vi "enable_by_name.vi"(8 "error in (no error)":errorcluster caption="错误输入（无错误）", 10 "name":string, 11 "MotorSystem 输入":refnum<class "MotorSystem.lvclass">) -> (0 "error out":errorcluster caption="错误输出", 3 "MotorSystem 输出":refnum<class "MotorSystem.lvclass">)   [LabVIEW 2016, in "MotionControl_UFO_3DOF.lvlib" / "MotorSystem.lvclass"]
uses:
  <userlib>/MotionControl_UFO_3DOF/MotorSystem/MotorSystem.lvclass
  <userlib>/MotionControl_UFO_3DOF/MotorSystem/MotorSystem.lvclass/MotorSystem.ctl
  <userlib>/MotionControl_UFO_3DOF/OneMotion/OneMotion.lvclass
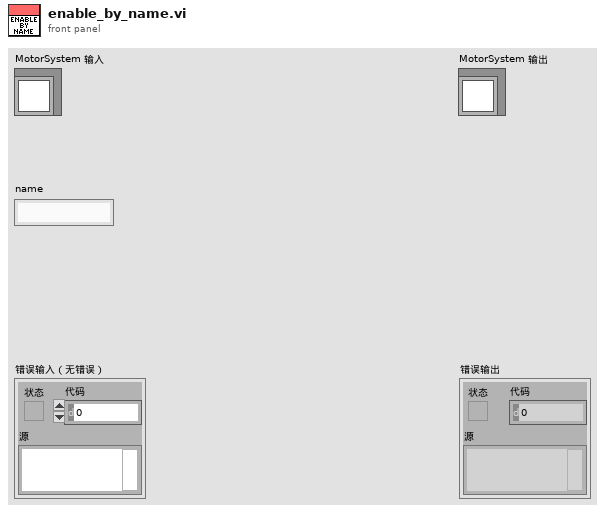
[diagram p1: front panel]
types:
  T1 = typedef "MotionControl_UFO_3DOF.lvlib/MotorSystem.lvclass/MotionCluster.ctl" = cluster{"OneMotion.lvclass":refnum<class "OneMotion.lvclass">, "connected?":bool, "default enabled?":bool, "enabled?":bool}
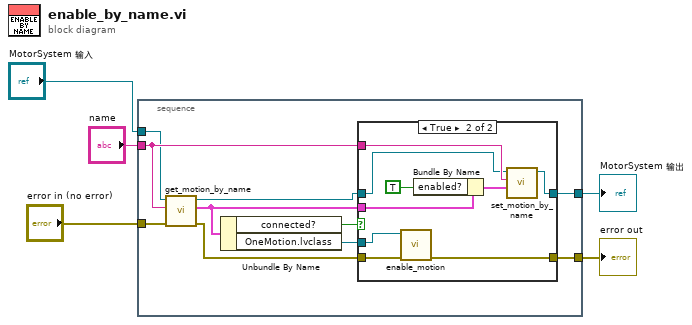
[diagram p0: block diagram]
diagram:
  n1 = stacked-sequence {
    tunnel: [w12] -> w5
    tunnel: [w7] -> w3
    tunnel: "MotorSystem 输入" -> [w8]
    tunnel: "error in (no error)" -> [w15]
    tunnel: "name" -> [w10]
    frame #0 {
      n2 = call <userlib>:"get_motion_by_name.vi"("error in (no error)"=w15, "name"=w10, "MotorSystem in"=w8) -> ("error out"=w13:errorcluster, "motion cluster"=w11:T1, "MotorSystem out"=w9:refnum<class "MotorSystem.lvclass">)  [unwired: 6 in]
      n3 = Unbundle By Name(w11) -> ("connected?"=w6:bool, "OneMotion.lvclass"=w14:refnum<class "OneMotion.lvclass">)
      n4 = case shown="True" w6 {
        tunnel: w14 -> [_ w26]
        tunnel: w13 -> [w16 w25]
        tunnel: [w16 w24] -> w12
        tunnel: w11 -> [_ w23]
        tunnel: w10 -> [_ w21]
        tunnel: w9 -> [w17 w20]
        tunnel: [w17 w18] -> w7
        frame False {
        }
        frame True {
          n5 = call <userlib>:"enable_motion.vi"("error in (no error)"=w25, "OneMotion 输入"=w26) -> ("error out"=w24:errorcluster)  [unwired: 8 in, 1 out]
          n6 = Bundle By Name(cluster=w23, "enabled?"=TRUE) -> (w19:T1)
          n7 = call <userlib>:"set_motion_by_name.vi"("簇"=w19, "name"=w21, "MotorSystem输入"=w20) -> ("MotorSystem输出"=w18:refnum<class "MotorSystem.lvclass">)  [unwired: 7 in, 1 out]
        }
      }
    }
  }
  "error out" <- w5
  "MotorSystem 输出" <- w3
